vi "Set Decimal Places.vi"(8 "error in (no error)":errorcluster, 9 "No. of Decimal Places":T1, 10 "Channel":T2, 11 "EPU452 in":refnum<class "EPU452.lvclass">) -> (0 "error out":errorcluster, 2 "Response":string, 3 "EPU452 out":refnum<class "EPU452.lvclass">)   [LabVIEW 2018, in "EPU452.lvclass"]
uses:
  EPU452.lvclass
  Controls/Channels.ctl
  Controls/Decimal Places.ctl
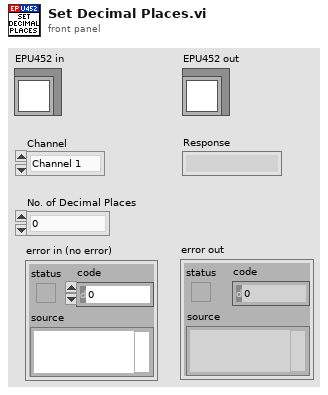
[diagram p1: front panel]
types:
  T1 = typedef "EPU452.lvclass/Decimal Places.ctl" = enum16{"0", "1", "2", "3", "4", "5", "6", "auto"}
  T2 = typedef "EPU452.lvclass/Channels.ctl" = enum16{"Channel 1", "Channel 2", "Channel 3", "Channel 4"}
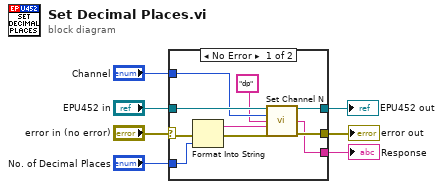
[diagram p0: block diagram]
diagram:
  n1 = case shown="No Error" "error in (no error)" {
    selector: "error in (no error)" -> [w11 w19]
    tunnel: [w13 w19] -> w6
    tunnel: [w14 w18] -> w4
    tunnel: "EPU452 in" -> [w17 w18]
    tunnel: "Channel" -> [w16 _]
    tunnel: "No. of Decimal Places" -> [w10 _]
    tunnel: [w9 _] -> w1
    frame No Error {
      n2 = Format Into String(error in=w11, w10) -> (resulting string=w8:string, error out=w12:errorcluster)  [unwired: 2 in]
      n3 = call "Set Channel N.vi"("EPU452 in"=w17, "Channel"=w16, "Function"="dp", "Argument/s"=w8, "error in (no error)"=w12) -> ("EPU452 out"=w14:refnum<class "EPU452.lvclass">, "Response"=w9:string, "error out"=w13:errorcluster)  [unwired: 8 in]
    }
    frame Error {
    }
  }
  "error out" <- w6
  "EPU452 out" <- w4
  "Response" <- w1
